vi "choose_single.vi"(9 "filetypes":string, 10 "Pfad in":path, 11 "deutsch?":bool) -> (3 "Pfad out":path)   [LabVIEW 2012]
uses:
  <vilib>/Utility/error.llb/DialogType.ctl
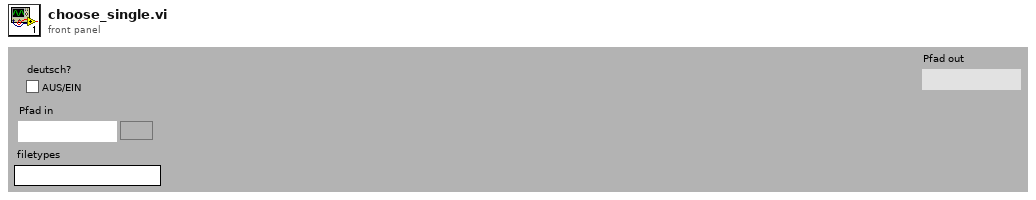
[diagram p1: front panel]
types:
  T1 = typedef "DialogType.ctl" = u16
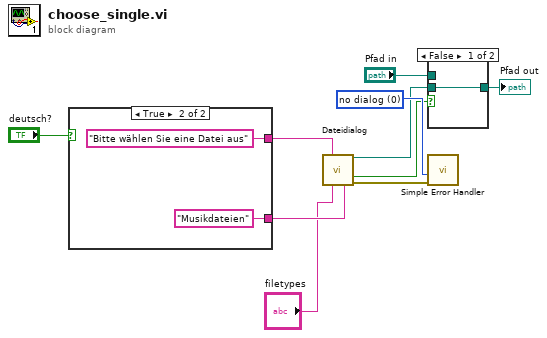
[diagram p0: block diagram]
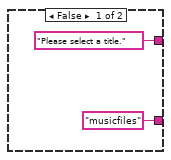
[diagram p3: hidden frame]
diagram:
  w6 = T1 0 items=["no dialog", "OK message", "continue or stop message", "OK message + warnings", "continue/stop + warnings"] ("type of dialog (OK msg:1)")
  n1 = case shown="True" "deutsch?" {
    tunnel: ["Please select a title." ("Eingabeaufforderung") "Bitte wählen Sie eine Datei aus" ("Eingabeaufforderung")] -> w10
    tunnel: ["musicfiles" "Musikdateien"] -> w9
    frame False {
    }
    frame True {
    }
  }
  n2 = call "Dateidialog"("prompt"=w10, "pattern (all files)"="filetypes", "pattern label"=w9) -> ("selected path"=w1:path, "cancelled"=w4:bool, "error out"=w5:errorcluster)  [unwired: 4 in, 6 out]
  n3 = case shown="False" w4 {
    tunnel: [w15 w16] -> w3
    tunnel: "Pfad in" -> [_ w16]
    tunnel: w1 -> [w15 _]
    frame False {
    }
    frame True {
    }
  }
  "Pfad out" <- w3
  n4 = call <vilib>:"Simple Error Handler.vi"("type of dialog (OK msg:1)"=w6, "error in (no error)"=w5) -> ()  [unwired: 1 in, 7 out]
